vi "生成CODMn data (子VI).vi"() -> (3 "data":T1)   [LabVIEW 2016, in "斯坦道CODMn.lvlib"]
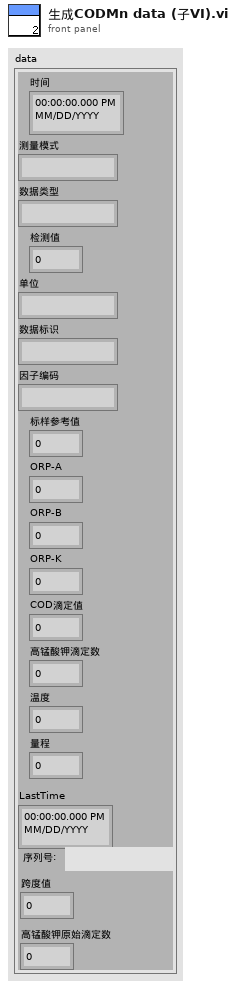
[diagram p1: front panel]
types:
  T1 = cluster{"时间":timestamp, "测量模式":string, "数据类型":string, "检测值":sgl, "单位":string, "数据标识":string, "因子编码":string, "标样参考值":sgl, "ORP-A":sgl, "ORP-B":sgl, "ORP-K":sgl, "COD滴定值":sgl, "高锰酸钾滴定数":sgl, "温度":sgl, "量程":sgl, "LastTime":timestamp, "序列号:":string, "跨度值":sgl, "高锰酸钾原始滴定数":sgl}
  T2 = cluster{"数组 2[0]":sgl, "数组 2[1]":sgl, "数组 2[2]":sgl, "数组 2[3]":sgl, "数组 2[4]":sgl, "数组 2[5]":sgl, "数组 2[6]":sgl, "数组 2[7]":sgl, "数组 2[8]":sgl, "数组 2[9]":sgl, "数组 2[10]":sgl, "数组 2[11]":sgl, "数组 2[12]":sgl, "数组 2[13]":sgl, "数组 2[14]":sgl, "数组 2[15]":sgl, "数组 2[16]":sgl, "数组 2[17]":sgl, "数组 2[18]":sgl, "数组 2[19]":sgl, "数组 2[20]":sgl, "数组 2[21]":sgl, "数组 2[22]":sgl, "数组 2[23]":sgl, "数组 2[24]":sgl, "数组 2[25]":sgl, "数组 2[26]":sgl, "数组 2[27]":sgl, "数组 2[28]":sgl, "数组 2[29]":sgl, "数组 2[30]":sgl, "数组 2[31]":sgl, "数组 2[32]":sgl, "数组 2[33]":sgl, "数组 2[34]":sgl, "数组 2[35]":sgl, "数组 2[36]":sgl, "数组 2[37]":sgl, "数组 2[38]":sgl, "数组 2[39]":sgl, "数组 2[40]":sgl, "数组 2[41]":sgl}
  T3 = cluster{"运行模式":enum16{"维护模式", "常规模式", "应急模式", "质控模式"}, "质控频次":enum16{"关闭", "每天", "星期一", "星期二", "星期三", "星期四", "星期五", "星期六", "星期日"}, "空白核查时间":u16, "跨度核查时间":u16, "测量间隔":u16}
  T4 = cluster{"测量量程":dbl, "测量精度":dbl, "测量间隔":dbl, "消解温度":dbl, "消解时长":dbl, "空白校准时间":timestamp, "曲线截距":dbl, "曲线斜率":dbl, "测量检出限":dbl, "测量信号值":dbl, "线性相关系数":dbl, "二次多项式系数":dbl, "标样校准时间":timestamp, "稀释倍数":dbl, "三项式系数":dbl, "空白标定系数":dbl, "量程系数":dbl, "F0/ORPA":dbl, "F1/ORPB":dbl, "F2/ORPK":dbl, "F3":dbl, "F4":dbl, "F5":dbl, "F6":dbl, "F7":dbl, "X0/滴定数":dbl, "量程":dbl}
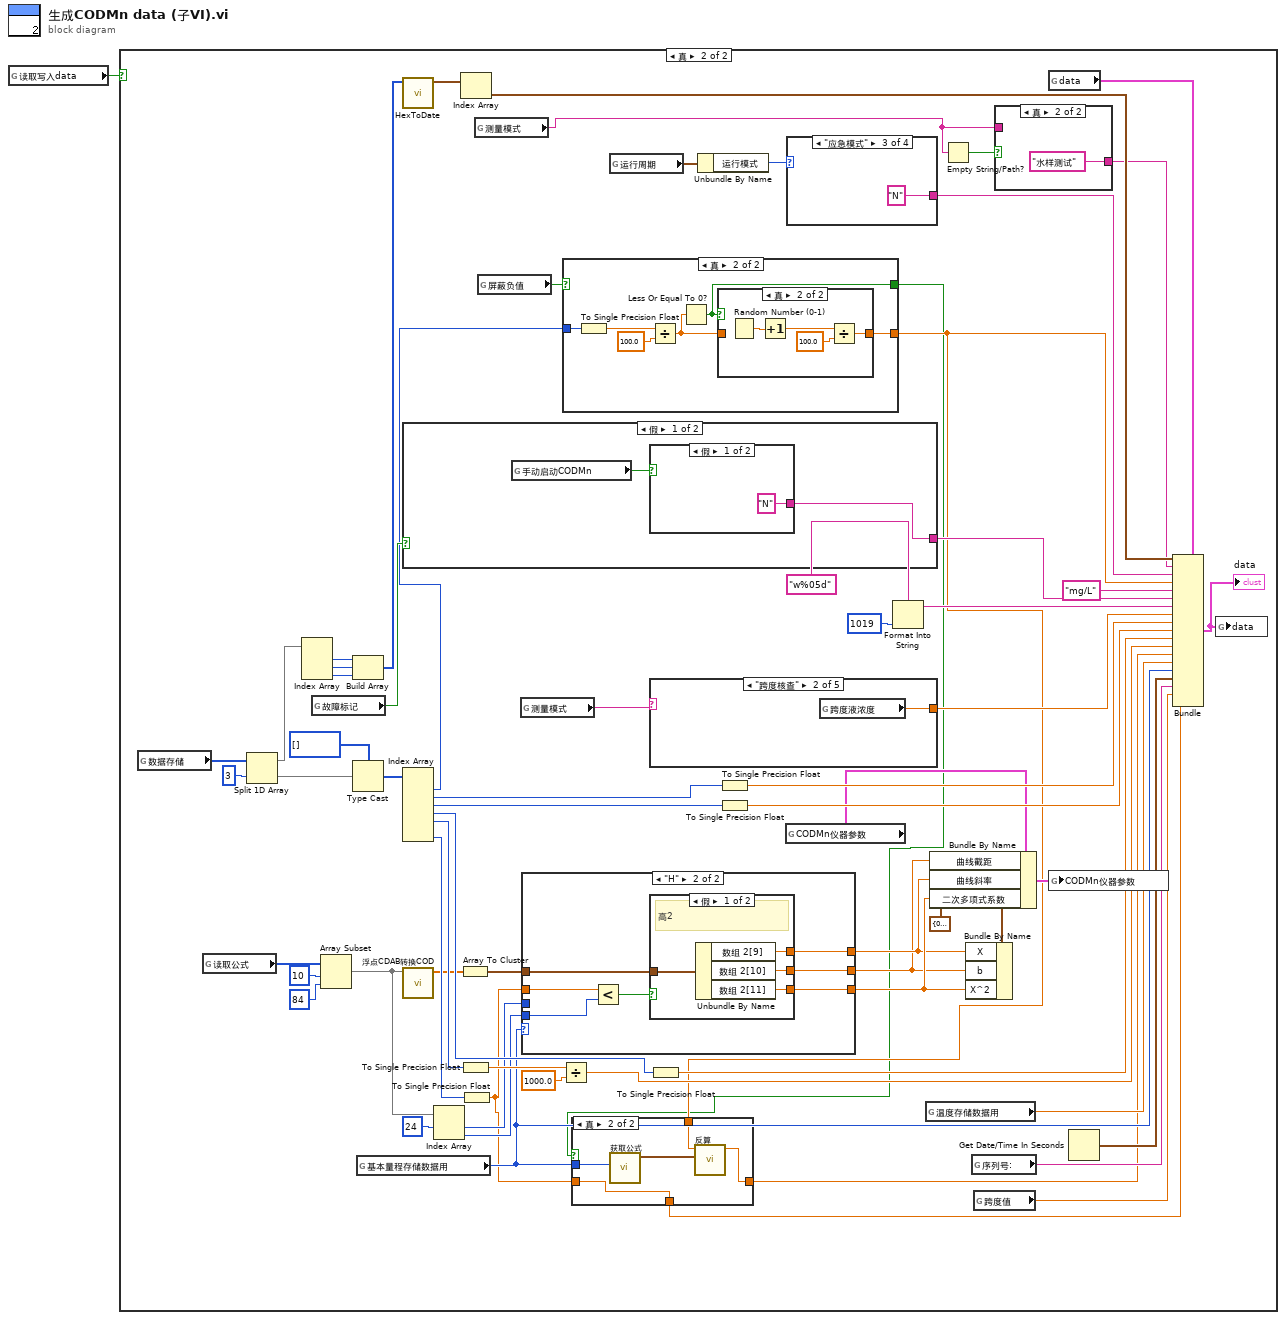
[diagram p0: block diagram]
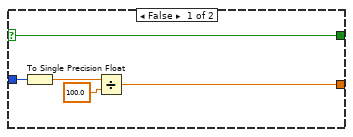
[diagram p4: hidden frame]
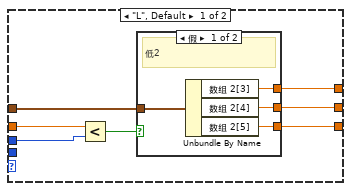
[diagram p7: hidden frame]
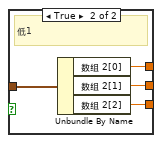
[diagram p8: hidden frame]
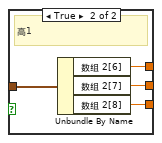
[diagram p9: hidden frame]
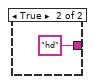
[diagram p10: hidden frame]
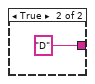
[diagram p11: hidden frame]
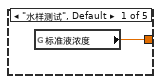
[diagram p12: hidden frame]
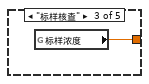
[diagram p13: hidden frame]
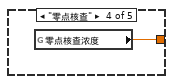
[diagram p14: hidden frame]
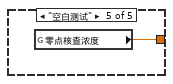
[diagram p15: hidden frame]
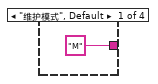
[diagram p16: hidden frame]
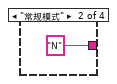
[diagram p17: hidden frame]
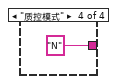
[diagram p18: hidden frame]
diagram:
  n1 = global read "COD内部交互全局.vi" "读取写入data"() -> (w1:bool)
  n2 = case shown="真" w1 {
    frame False {
    }
    frame True {
      n3 = global read "COD内部交互全局.vi" "数据存储"() -> (w37:u16[])
      n4 = global read "COD内部交互全局.vi" "读取公式"() -> (w23:u16[])
      n5 = Split 1D Array(array=w37, index=3 ("索引")) -> (first subarray=w41:u16[], second subarray=w36:u16[])
      n6 = Index Array(array=w41) -> (element #1=w43:u16, element #2=w44:u16, element #3=w45:u16)  [unwired: 3 in]
      n7 = global read "COD内部交互全局.vi" "故障标记"() -> (w67:bool)
      n8 = Array Subset(array=w23, index=10 ("索引"), length=84 ("长度")) -> (w19:u16[])
      n9 = Build Array(w43, w44, w45) -> (w46:u16[])
      n10 = Type Cast(type=i16[] [], x=w36) -> (*(type *) &x=w35:i16[])
      n11 = global read "COD内部交互全局.vi" "基本量程存储数据用"() -> (w12:enum16{"L", "H", "AUTO"})
      n12 = call "HexToDate.vi"("数组"=w46) -> ("DATE"=w42:timestamp[])  [unwired: 10 in]
      n13 = case shown="假" w67 {
        tunnel: [w123 "D" ("数据标识")] -> w60
        frame False {
          n14 = global read "CODMN外部API.vi" "手动启动CODMn"() -> (w122:bool)
          n15 = case shown="假" w122 {
            tunnel: ["N" ("数据标识") "hd" ("数据标识")] -> w123
            frame False {
            }
            frame True {
            }
          }
        }
        frame True {
        }
      }
      n16 = Index Array(array=w35) -> (element #1=w63:i16, element #2=w47:i16, element #3=w48:i16, element #4=w49:i16, element #5=w50:i16, element #7=w65:i16)  [unwired: 7 in, 1 out]
      n17 = call "浮点CDAB转换COD.vi"("数组"=w19) -> ("数组 2"=w22:sgl[])  [unwired: 10 in]
      n18 = Index Array(array=w19, index #1=24 ("索引")) -> (element #1=w25:u16, element #2=w26:u16)  [unwired: 1 in]
      n19 = Array To Cluster(array=w22) -> (cluster=w24:T2)
      n20 = Index Array(array=w42) -> (element=w34:timestamp)  [unwired: 1 in]
      n21 = To Single Precision Float(number=w50) -> (single precision float=w53:sgl)
      n22 = To Single Precision Float(number=w65) -> (single precision float=w9:sgl)
      n23 = global read "CODMn断电保存全局变量.vi" "测量模式"() -> (w3:string)
      n24 = global read "CODMn断电保存全局变量.vi" "屏蔽负值"() -> (w7:bool)
      n25 = global read "CODMn断电保存全局变量.vi" "测量模式"() -> (w2:string)
      n26 = case shown="\"H\"" w12 {
        tunnel: w24 -> [w95 w112]
        tunnel: w25 -> [w97 _]
        tunnel: w26 -> [_ w110]
        tunnel: w9 -> [w98 w111]
        tunnel: [w94 w109] -> w14
        tunnel: [w93 w108] -> w13
        tunnel: [w92 w107] -> w15
        frame "L", Default {
          n27 = Less?(x=w98, y=w97) -> (x < y?=w96:bool)
          n28 = case shown="假" w96 {
            tunnel: w95 -> [w102 w106]
            tunnel: [w101 w105] -> w94
            tunnel: [w100 w104] -> w93
            tunnel: [w99 w103] -> w92
            frame False {
              # "低2"
              n29 = Unbundle By Name(w102) -> ("数组 2[3]"=w101:sgl, "数组 2[4]"=w100:sgl, "数组 2[5]"=w99:sgl)
            }
            frame True {
              # "低1"
              n30 = Unbundle By Name(w106) -> ("数组 2[0]"=w105:sgl, "数组 2[1]"=w104:sgl, "数组 2[2]"=w103:sgl)
            }
          }
        }
        frame "H" {
          n31 = Less?(x=w111, y=w110) -> (x < y?=w113:bool)
          n32 = case shown="假" w113 {
            tunnel: w112 -> [w117 w121]
            tunnel: [w116 w120] -> w109
            tunnel: [w115 w119] -> w108
            tunnel: [w114 w118] -> w107
            frame False {
              # "高2"
              n33 = Unbundle By Name(w117) -> ("数组 2[9]"=w116:sgl, "数组 2[10]"=w115:sgl, "数组 2[11]"=w114:sgl)
            }
            frame True {
              # "高1"
              n34 = Unbundle By Name(w121) -> ("数组 2[6]"=w120:sgl, "数组 2[7]"=w119:sgl, "数组 2[8]"=w118:sgl)
            }
          }
        }
      }
      n35 = Divide(x=w53, y=sgl 1000.0) -> (x/y=w55:sgl)
      n36 = case shown="真" w7 {
        selector: w7 -> [w70 _]
        tunnel: w63 -> [w72 w77]
        tunnel: [w71 w80] -> w11
        tunnel: [w70 w76] -> w8
        frame False {
          n37 = To Single Precision Float(number=w72) -> (single precision float=w74:sgl)
          n38 = Divide(x=w74, y=sgl 100.0) -> (x/y=w71:sgl)
        }
        frame True {
          n39 = To Single Precision Float(number=w77) -> (single precision float=w78:sgl)
          n40 = Divide(x=w78, y=sgl 100.0) -> (x/y=w75:sgl)
          n41 = Less Or Equal To 0?(x=w75) -> (x <= 0?=w76:bool)
          n42 = case shown="真" w76 {
            tunnel: [w81 w85] -> w80
            tunnel: w75 -> [w81 _]
            frame False {
            }
            frame True {
              n43 = Random Number (0-1)() -> (number: 0 to 1=w84:dbl)
              n44 = Increment(x=w84) -> (x+1=w82:dbl)
              n45 = Divide(x=w82, y=sgl 100.0) -> (x/y=w85:dbl)
            }
          }
        }
      }
      n46 = case shown="真" w8 {
        tunnel: w12 -> [_ w90]
        tunnel: w11 -> [_ w89]
        tunnel: [w86 w88] -> w10
        tunnel: w9 -> [w86 w87]
        tunnel: [w86 w87] -> w6
        frame False {
        }
        frame True {
          n47 = call "获取公式.vi"("量程选择"=w90) -> ("方程系数"=w91:cluster{"X^2":dbl, "K":dbl, "b":dbl})  [unwired: 9 in, 1 out]
          n48 = call "反算.vi"("公式"=w91, "监测值"=w89) -> ("信号值"=w88:dbl)  [unwired: 8 in, 1 out]
        }
      }
      n49 = global read "CODMn断电保存全局变量.vi" "运行周期"() -> (w31:T3)
      n50 = case shown="\"跨度核查\"" w2 {
        tunnel: [w127 w128 w129 w130 w131] -> w64
        frame "水样测试", Default {
          n51 = global read "COD浓度全局变量.vi" "标准液浓度"() -> (w127:dbl)
        }
        frame "跨度核查" {
          n52 = global read "CODMn断电保存全局变量.vi" "跨度液浓度"() -> (w128:dbl)
        }
        frame "标样核查" {
          n53 = global read "CODMn断电保存全局变量.vi" "标样浓度"() -> (w129:dbl)
        }
        frame "零点核查" {
          n54 = global read "CODMn断电保存全局变量.vi" "零点核查浓度"() -> (w130:dbl)
        }
        frame "空白测试" {
          n55 = global read "CODMn断电保存全局变量.vi" "零点核查浓度"() -> (w131:dbl)
        }
      }
      n56 = To Single Precision Float(number=w49) -> (single precision float=w56:sgl)
      n57 = Unbundle By Name(w31) -> ("运行模式"=w30:enum16{"维护模式", "常规模式", "应急模式", "质控模式"})
      n58 = To Single Precision Float(number=w47) -> (single precision float=w58:sgl)
      n59 = To Single Precision Float(number=w48) -> (single precision float=w57:sgl)
      n60 = global read "CODMn断电保存全局变量.vi" "CODMn仪器参数"() -> (w17:T4)
      n61 = case shown="\"应急模式\"" w30 {
        tunnel: ["M" ("单位") "N" ("单位") "N" ("单位") "N" ("单位")] -> w62
        frame "维护模式", Default {
        }
        frame "常规模式" {
        }
        frame "应急模式" {
        }
        frame "质控模式" {
        }
      }
      n62 = Format Into String(format string="w%05d" ("格式字符串"), u32 1019 ("因子编码")) -> (resulting string=w59:string)  [unwired: 2 in, 1 out]
      n63 = global read "COD内部交互全局.vi" "温度存储数据用"() -> (w66:dbl)
      n64 = Bundle By Name(cluster=w17, "曲线截距"=w13, "曲线斜率"=w14, "二次多项式系数"=w15) -> (w16:T4)
      n65 = Empty String/Path?(string/path=w3) -> (empty?=w5:bool)
      n66 = Bundle By Name(cluster=cluster{"X":dbl, "b":dbl, "X^2":dbl} {"X"=0.0, "b"=0.0, "X^2"=0.0} ("方程系数"), "X"=w14, "b"=w13, "X^2"=w15) -> ()  [unwired: 1 out]
      n67 = global read "COD内部交互全局.vi" "序列号:"() -> (w33:string)
      n68 = global read "CODMn断电保存全局变量.vi" "跨度值"() -> (w28:dbl)
      n69 = case shown="真" w5 {
        tunnel: [w68 "水样测试" ("测量模式")] -> w4
        tunnel: w3 -> [w68 _]
        frame False {
        }
        frame True {
        }
      }
      n70 = global read "COD内部交互全局.vi" "data"() -> (w29:T1)
      n71 = global write "CODMn断电保存全局变量.vi" "CODMn仪器参数"(w16) -> ()
      n72 = Get Date/Time In Seconds() -> (seconds since 1Jan1904=w39:timestamp)
      n73 = Bundle(cluster=w29, "时间"=w34, "测量模式"=w4, "数据类型"=w62, "检测值"=w11, "单位"="mg/L", "数据标识"=w60, "因子编码"=w59, "标样参考值"=w64, "ORP-A"=w58, "ORP-B"=w57, "ORP-K"=w56, "COD滴定值"=w55, "高锰酸钾滴定数"=w10, "温度"=w66, "量程"=w12, "LastTime"=w39, "序列号:"=w33, "跨度值"=w28, "高锰酸钾原始滴定数"=w6) -> (w32:T1)
      "data" <- w32
      n74 = global write "COD内部交互全局.vi" "data"(w32) -> ()
    }
  }
